vi "Async Stop video from CamServer (for web monitoring).vi"() -> (0 "Error out":errorcluster)   [LabVIEW 2016]
uses:
  Globals/CamServer global.vi
panel:
  # "PN 21/08/15"
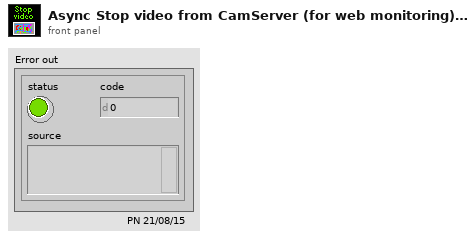
[diagram p1: front panel]
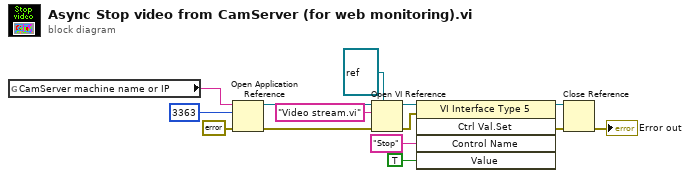
[diagram p0: block diagram]
diagram:
  n1 = global read "CamServer global.vi" "CamServer machine name or IP"() -> (w1:string)
  n2 = Open Application Reference(8:errorcluster {"status"=FALSE, "code"=0, "source"=""} ("error in (no error)"), 10:u16 3363 ("port"), 11:w1) -> (0:w11:errorcluster, 3:w12:refnum<vi>)  [unwired: 1 in]
  n3 = Open VI Reference(type specifier VI Refnum (for type only)=refnum<vi> refnum, application reference (local)=w12, vi path="Video stream.vi" ("machine name"), error in (no error)=w11) -> (vi reference=w8:refnum<vi>, error out=w5:errorcluster)  [unwired: 2 in]
  n4 = invoke class="VI Interface Type 5" method="Ctrl Val.Set"(reference=w8, error in=w5, "Control Name"="Stop", "Value"=TRUE) -> (reference out=w7:refnum<vi>, error out=w4:errorcluster)  [unwired: 1 in, 3 out]
  n5 = Close Reference(reference=w7, error in (no error)=w4) -> (error out=→"Error out":errorcluster)
